vi "Teleop_Calc_Twist.vi"(11 "Teleop Local Data in":T1) -> (3 "Teleop Local Data out":T1)   [LabVIEW 2016]
uses:
  Typedefs/typedef_cluster_Teleop Local Data.ctl
  Typedefs/typedef_enum_Joystick Buttons.ctl
  Typedefs/typedef_enum_Joystick Axes.ctl
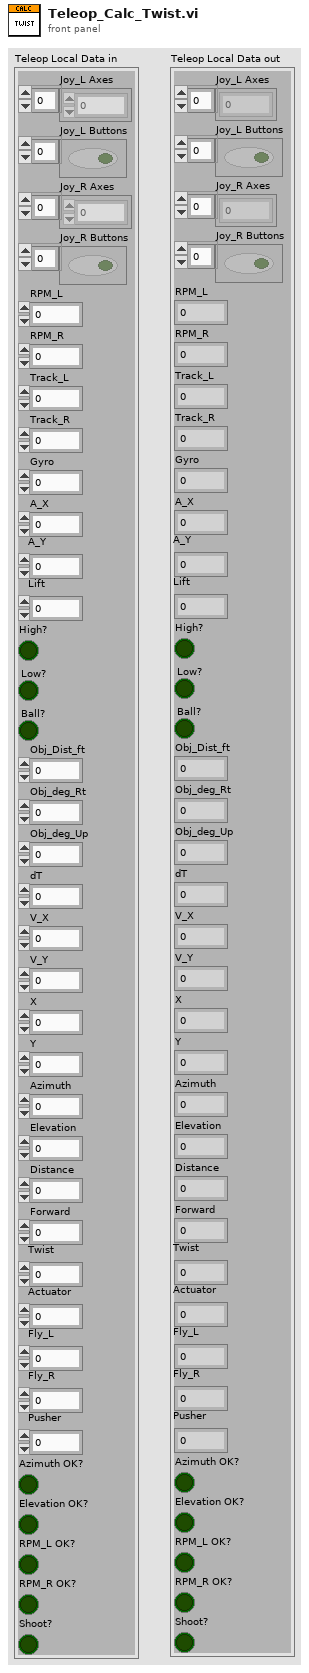
[diagram p1: front panel]
types:
  T1 = typedef "typedef_cluster_Teleop Local Data.ctl" = cluster{"Joy_L Axes":dbl[], "Joy_L Buttons":bool[], "Joy_R Axes":dbl[], "Joy_R Buttons":bool[], "RPM_L":dbl, "RPM_R":dbl, "Track_L":dbl, "Track_R":dbl, "Gyro":dbl, "A_X":dbl, "A_Y":dbl, "Lift":dbl, "High?":bool, "Low?":bool, "Ball?":bool, "Obj_Dist_ft":dbl, "Obj_deg_Rt":dbl, "Obj_deg_Up":dbl, "dT":dbl, "V_X":dbl, "V_Y":dbl, "X":dbl, "Y":dbl, "Azimuth":dbl, "Elevation":dbl, "Distance":dbl, "Forward":dbl, "Twist":dbl, "Actuator":dbl, "Fly_L":dbl, "Fly_R":dbl, "Pusher":dbl, "Azimuth OK?":bool, "Elevation OK?":bool, "RPM_L OK?":bool, "RPM_R OK?":bool, "Shoot?":bool}
  T2 = typedef "typedef_enum_Joystick Axes.ctl" = enum16{"LeftRight", "ForeBack", "Twist", "Throttle"}
  T3 = typedef "typedef_enum_Joystick Buttons.ctl" = enum16{"Trigger", "Thumb", "Top3", "Top4", "Top5", "Top6", "Low7", "Low8", "Low9", "Low10", "Low11", "Low12", "Hat0", "Hat1", "Hat2", "Hat3", "Hat4", "Hat5", "Hat6", "Hat7", "Hat8"}
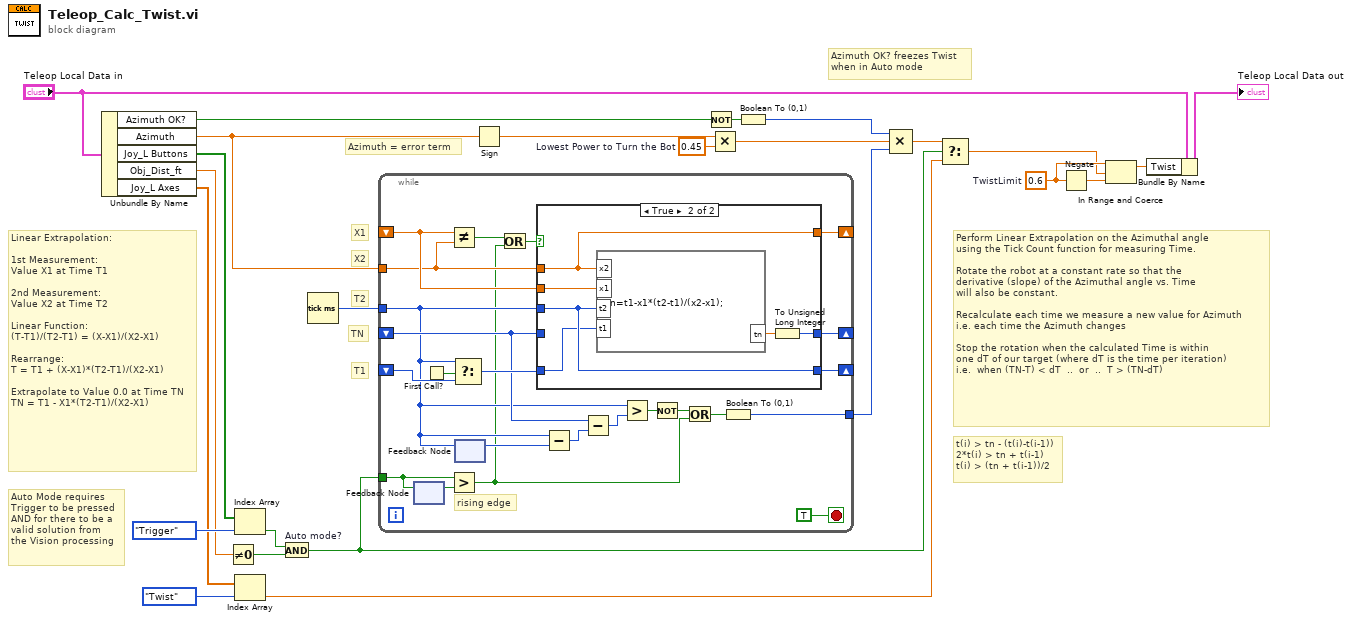
[diagram p0: block diagram]
diagram:
  w5 = 0.45  # Lowest Power to Turn the Bot
  w13 = 0.6  # TwistLimit
  # "Auto Mode requires\nTrigger to be pressed\nAND for there to be a\nvalid solution from\nthe Vision processing"
  # "T2"
  # "X2"
  # "X1"
  # "T1"
  # "TN"
  # "t(i) > tn - (t(i)-t(i-1))\n2*t(i) > tn + t(i-1)\nt(i) > (tn + t(i-1))/2"
  # "Perform Linear Extrapolation on the Azimuthal angle\nusing the Tick Count function for measuring Time.\n\nRotate the robot at a constant rate so that the\nderivative (slope) of the Azimuthal angle vs. Time \nwill also be constant.\n\nRecalculate each time we measure a new value for Azimuth\ni.e. each time the Azimuth changes\n\nStop the rotation when the calculated Time is within\none dT of our target (where dT is the time per iteration)\ni.e.  when (TN-T) < dT  ..  or  ..  T > (TN-dT)"
  # "Linear Extrapolation:\n\n1st Measurement:\nValue X1 at Time T1\n\n2nd Measurement:\nValue X2 at Time T2\n\nLinear Function:\n(T-T1)/(T2-T1) = (X-X1)/(X2-X1)\n\nRearrange:\nT = T1 + (X-X1)*(T2-T1)/(X2-X1)\n\nExtrapolate to Value 0.0 at Time TN\nTN = T1 - X1*(T2-T1)/(X2-X1)"
  # "Azimuth OK? freezes Twist\nwhen in Auto mode"
  # "Azimuth = error term"
  n1 = Unbundle By Name("Teleop Local Data in") -> ("Azimuth OK?"=w17:bool, "Azimuth"=w4:dbl, "Joy_L Buttons"=w20:bool[], "Obj_Dist_ft"=w19:dbl, "Joy_L Axes"=w9:dbl[])
  n2 = Not Equal To 0?(x=w19) -> (x != 0?=w23:bool)
  n3 = Index Array(array=w20, index=typedef_enum_Joystick_Buttons."Trigger" ("Joystick Buttons")) -> (element=w22:bool)
  n4 = Index Array(array=w9, index=typedef_enum_Joystick_Axes."Twist" ("Joystick Axes")) -> (element=w10:dbl)
  n5 = And "Auto mode?"(x=w22, y=w23) -> (x .and. y?=w1:bool)
  n6 = Tick Count (ms)() -> (millisecond timer value=w2:u32)
  n7 = while {
    tunnel: w4 -> [w31]
    shift-right: [w48] -> _
    shift-left: _ -> [w45]
    shift-right: [w47] -> _
    shift-left: _ -> [w40]
    tunnel: [w37] -> w3
    shift-right: [w33] -> _
    shift-left: _ -> [w32]
    tunnel: w2 -> [w30]
    tunnel: w1 -> [w27]
    stop <- TRUE stop-if-true
    # "rising edge"
    n8 = feedback #1() -> (w29:bool)  [unwired: 1 in]
    n9 = feedback-in #1(w27) -> ()
    n10 = First Call?() -> (First Call?: T/F=w46:bool)
    n11 = Not Equal?(x=w32, y=w31) -> (x != y?=w34:bool)
    n12 = Greater?(x=w27, y=w29) -> (0:w28:bool)
    n13 = Select(t=w30, s=w46, f=w45) -> (s? t:f=w44:u32)
    n14 = feedback #2() -> (w41:u32)  [unwired: 1 in]
    n15 = feedback-in #2(w30) -> ()
    n16 = Or(x=w34, y=w28) -> (x .or. y?=w35:bool)
    n17 = case shown="True" w35 {
      tunnel: w31 -> [_ w53]
      tunnel: w30 -> [_ w57]
      tunnel: [w51 w57] -> w48
      tunnel: w44 -> [w51 w56]
      tunnel: [w50 w54] -> w47
      tunnel: w40 -> [w50 _]
      tunnel: [w49 w53] -> w33
      tunnel: w32 -> [w49 w52]
      frame False {
      }
      frame True {
        n18 = formula code="tn=t1-x1*(t2-t1)/(x2-x1);"("x2"=w53, "x1"=w52, "t2"=w57, "t1"=w56) -> ("tn"=w55:dbl)
        n19 = To Unsigned Long Integer(number=w55) -> (unsigned 32bit integer=w54:u32)
      }
    }
    n20 = Subtract(x=w30, y=w41) -> (x-y=w42:u32)
    n21 = Subtract(x=w40, y=w42) -> (x-y=w43:u32)
    n22 = Greater?(x=w30, y=w43) -> (0:w39:bool)
    n23 = Not(x=w39) -> (.not. x?=w38:bool)
    n24 = Or(x=w38, y=w28) -> (x .or. y?=w36:bool)
    n25 = Boolean To (0,1)(Boolean=w36) -> (0, 1=w37:i16)
  }
  n26 = Sign(1:w4) -> (0:w6:dbl)
  n27 = Not(x=w17) -> (.not. x?=w16:bool)
  n28 = Multiply(x=w6, y=w5) -> (x*y=w7:dbl)
  n29 = Boolean To (0,1)(Boolean=w16) -> (0, 1=w15:i16)
  n30 = Compound Arithmetic op=MULTIPLY(w15, w7, w3) -> (w8:dbl)
  n31 = Select(t=w8, s=w1, f=w10) -> (s? t:f=w11:dbl)
  n32 = Negate(x=w13) -> (-x=w12:dbl)
  n33 = In Range and Coerce(upper limit=w13, x=w11, lower limit=w12) -> (coerced(x)=w14:dbl)  [unwired: 1 out]
  n34 = Bundle By Name(cluster="Teleop Local Data in", "Twist"=w14) -> (→"Teleop Local Data out":T1)
